vi "ActorDatabase-PerformUpdate.vi"(7 "Payload From Actor":string, 8 "error in (no error)":errorcluster, 11 "Database-Actor in":refnum<class "PartCertDatabase-Actor.lvclass">) -> (0 "error out":errorcluster, 3 "Database-Actor out":refnum<class "PartCertDatabase-Actor.lvclass">, 5 "Payload to Actor":string)   [LabVIEW 2013, in "PartCertDatabase-Actor.lvclass"]
uses:
  PartCertDatabase-Actor.lvclass
  Reuse Library/Database API/PartCertDatabase-API.lvclass
  ftw-dataflow/Core/utils/CodeGen/JSON Deserialize/FTW-JSON-Deserialize.xnode
  <vilib>/addons/database/Auxilliary.llb/DB Tools DataTypes.ctl
  <vilib>/addons/database/NI_Database_API.lvlib
  ftw-dataflow/Core/src/Reflection/FTW-Reflection-Type.vi
  ftw-dataflow/Core/src/JSON/FTW-JSON-Core-GetFlattenedValue.vi
  ftw-dataflow/Core/src/JSON/FTW-JSON-Core-LibraryFilepath.vi
  ftw-dataflow/Core/src/JSON/FTW-JSON-Core-LibraryError.vi
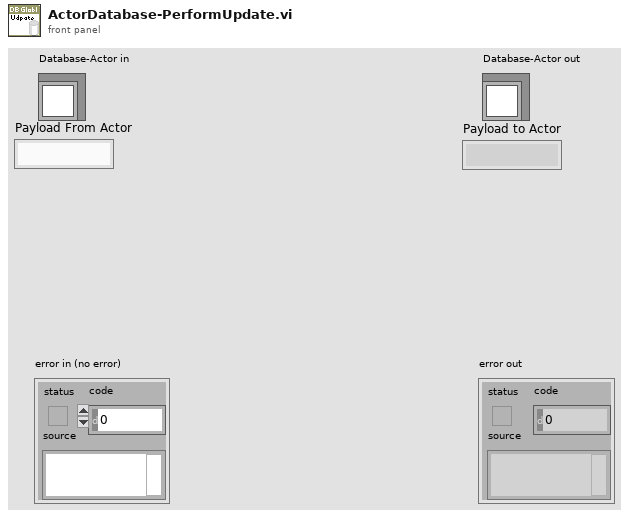
[diagram p1: front panel]
types:
  T1 = typedef "NI_Database_API.lvlib/DB Tools DataTypes.ctl" = enum16{"String", "Long (I32)", "Single (SGL)", "Double (DBL)", "Date/Time", "Binary"}
  T2 = cluster{"name":string, "database data type":T1, "defined size":i32}[]
  T3 = cluster{"Table":string, "SQL Statement":string, "Update All":bool, "Payload":string, "Column Number":i32, "Datatype":i32}
  T4 = cluster{"Path for Picture Material":path, "Path for Picture Material 2":path, "Path for Picture Material 3":path, "Path for Picture Material 4":path, "Path for Picture Material 5":path, "Path for Picture Material 6":path, "Path for Picture Material 7":path, "Get Material Instruction":string}[]
  T5 = cluster{"[0]":string, "[1]":string, "[2]":string, "[3]":string, "[4]":string, "[5]":string, "[6]":string, "[7]":string, "[8]":string}
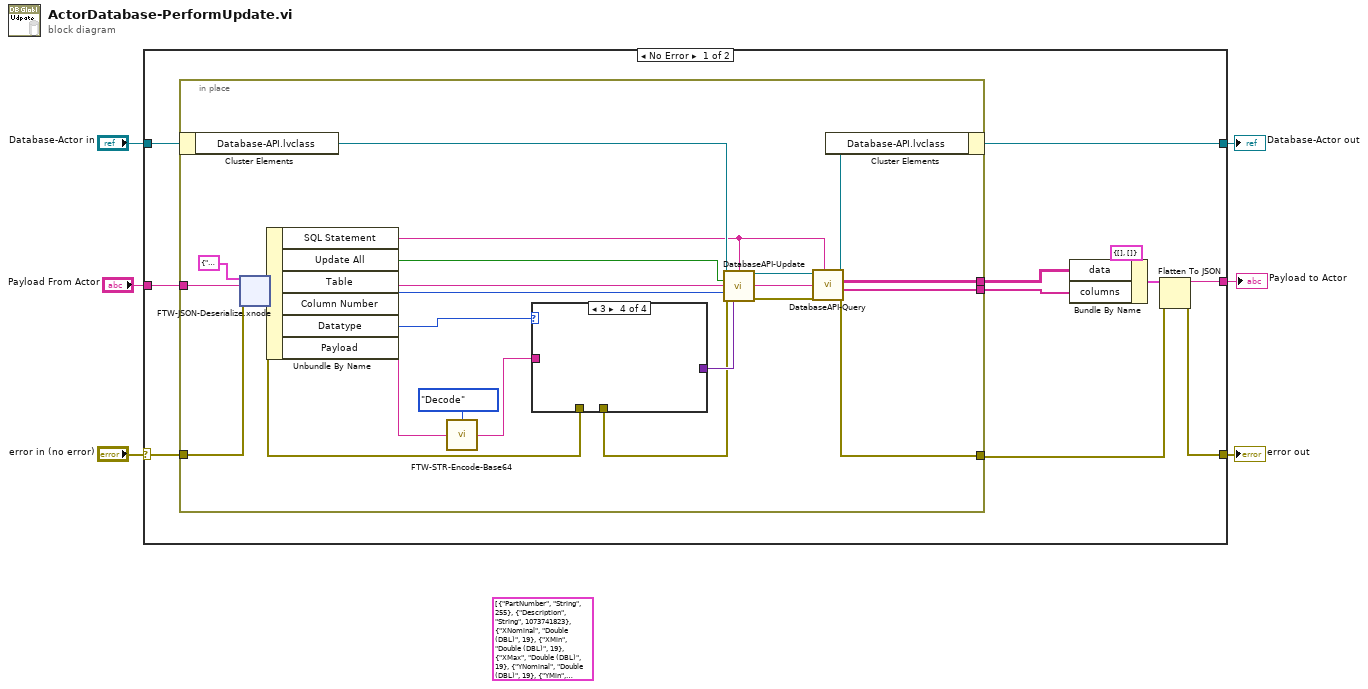
[diagram p0: block diagram]
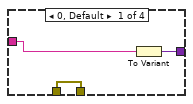
[diagram p2: hidden frame]
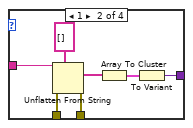
[diagram p3: hidden frame]
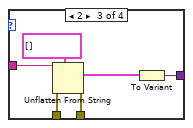
[diagram p4: hidden frame]
diagram:
  (unwired) T2 [{"name"="PartNumber", "database data type"=enum."String", "defined size"=255}, {"name"="Description", "database data type"=enum."String", "defined size"=1073741823}, {"name"="XNominal", "database data type"=enum."Double (DBL)", "defined size"=19}, {"name"="XMin", "database data type"=enum."Double (DBL)", "defined size"=19}, {"name"="XMax", "database data type"=enum."Double (DBL)", "defined size"=19}, {"name"="YNominal", "database data type"=enum."Double (DBL)", "defined size"=19}, {"name"="YMin", "database data type"=enum."Double (DBL)", "defined size"=19}, {"name"="YMax", "database data type"=enum."Double (DBL)", "defined size"=19}, {"name"="ZNominal", "database data type"=enum."Double (DBL)", "defined size"=19}, {"name"="ZMin", "database data type"=enum."Double (DBL)", "defined size"=19}, {"name"="ZMax", "database data type"=enum."Double (DBL)", "defined size"=19}, {"name"="DIANominal", "database data type"=enum."Double (DBL)", "defined size"=19}, {"name"="DIAMin", "database data type"=enum."Double (DBL)", "defined size"=19}, {"name"="DIAMax", "database data type"=enum."Double (DBL)", "defined size"=19}, {"name"="HarndessMin", "database data type"=enum."Double (DBL)", "defined size"=19}, {"name"="HardnessMax", "database data type"=enum."Double (DBL)", "defined size"=19}, {"name"="TackMin", "database data type"=enum."Double (DBL)", "defined size"=19}, {"name"="TackMax", "database data type"=enum."Double (DBL)", "defined size"=19}, {"name"="AverySmlBackLabel", "database data type"=enum."String", "defined size"=10}, {"name"="AverySmlFrontLabel", "database data type"=enum."String", "defined size"=10}, {"name"="AveryMedBackLabel", "database data type"=enum."String", "defined size"=10}, {"name"="AveryMedFrontLabel", "database data type"=enum."String", "defined size"=10}, {"name"="BagLabel", "database data type"=enum."String", "defined size"=10}, {"name"="ContainerLabel", "database data type"=enum."String", "defined size"=10}, {"name"="NoLabels", "database data type"=enum."String", "defined size"=10}, {"name"="CustomLabel", "database data type"=enum."String", "defined size"=10}, {"name"="CutPart", "database data type"=enum."String", "defined size"=10}] ("column information")
  n1 = case shown="No Error" "error in (no error)" {
    selector: "error in (no error)" -> [w15 w91]
    tunnel: [w8 w91] -> w5
    tunnel: [w16 w90] -> w3
    tunnel: "Database-Actor in" -> [w17 w90]
    tunnel: "Payload From Actor" -> [w14 _]
    tunnel: [w7 _] -> w1
    frame No Error {
      n2 = in-place {
        in-place-border: w15 -> [w38]
        in-place-border: [w30] -> w9
        in-place-border: w14 -> [w20]
        in-place-border: [w19] -> w11
        in-place-border: [w18] -> w10
        n3 = in-place-cluster #1(w17) -> ("Database-API.lvclass"=w39:refnum<class "PartCertDatabase-API.lvclass">)
        n4 = xnode "FTW-JSON-Deserialize.xnode"("Type and Defaults"=T3 {"Table"="", "SQL Statement"="", "Update All"=FALSE, "Payload"="", "Column Number"=0, "Datatype"=0} ("output cluster"), "JSON String"=w20, "error in"=w38) -> ("Values"=w21:T3, "error out"=w26:errorcluster)
        n5 = Unbundle By Name(w21) -> ("SQL Statement"=w34:string, "Update All"=w37:bool, "Table"=w32:string, "Column Number"=w24:i32, "Datatype"=w28:i32, "Payload"=w27:string)
        n6 = call "FTW-STR-Encode-Base64.vi"("Input"=w27, "Direction"=enum16{"Encode", "Decode"}."Decode") -> ("Output"=w23:string)
        n7 = case shown="3" w28 {
          tunnel: w23 -> [w41 w48 w55 _]
          tunnel: [w42 w45 w54 _] -> w35
          tunnel: w26 -> [w40 w44 w53 _]
          tunnel: [w40 w43 w52 _] -> w25
          frame 0, Default {
            n8 = To Variant(anything=w41) -> (Variant=w42:variant)
          }
          frame 1 {
            n9 = Unflatten From String(type=string[] [], binary string=w48, error in (no error)=w44) -> (value=w47:string[], error out=w43:errorcluster)  [unwired: 2 in, 1 out]
            n10 = Array To Cluster(array=w47) -> (cluster=w46:T5)
            n11 = To Variant(anything=w46) -> (Variant=w45:variant)
          }
          frame 2 {
            n12 = Unflatten From String(type=T4 [] ("appended array"), binary string=w55, error in (no error)=w53) -> (value=w50:T4, error out=w52:errorcluster)  [unwired: 2 in, 1 out]
            n13 = To Variant(anything=w50) -> (Variant=w54:variant)
          }
          frame 3 {
          }
        }
        n14 = call "DatabaseAPI-Update.vi"("Database-API in"=w39, "data"=w35, "Where Statement"=w34, "Update All"=w37, "Table"=w32, "Column Number"=w24, "error in (no error)"=w25) -> ("Database-API out"=w33:refnum<class "PartCertDatabase-API.lvclass">, "error out"=w31:errorcluster)  [unwired: 7 in]
        n15 = call "DatabaseAPI-Query.vi"("optional clause"=w34, "error in (no error)"=w31, "Table"=w32, "Database-API in"=w33) -> ("error out"=w30:errorcluster, "columns"=w18:string[], "data"=w19:string[][], "Database-API out"=w29:refnum<class "PartCertDatabase-API.lvclass">)  [unwired: 4 in]
        n16 = in-place-cluster #1("Database-API.lvclass"=w29) -> (w16:refnum<class "PartCertDatabase-Actor.lvclass">)
      }
      n17 = Bundle By Name(cluster=cluster{"data":string[][], "columns":string[]} {"data"=[], "columns"=[]}, "data"=w11, "columns"=w10) -> (w12:cluster{"data":string[][], "columns":string[]})
      n18 = Flatten To JSON(anything=w12, error in (no error)=w9) -> (JSON string=w7:string, 11:w8:errorcluster)  [unwired: 1 in]
    }
    frame Error {
    }
  }
  "error out" <- w5
  "Database-Actor out" <- w3
  "Payload to Actor" <- w1
